vi "autonSample.vi"(0 "Auton Array":dbl[][](array[numeric]), 5 "MeasuredHeading":dbl, 9 "EncoderDistance":dbl) -> (4 "Left Drive":dbl(knob) scale=-1.0..1.0, 6 "Right Drive":dbl(knob) scale=-1.0..1.0, 10 "Turret Rotation":dbl, 14 "Feeder motor":dbl, 15 "Shooter motor output":dbl)   [LabVIEW 2011]
uses:
  Robot Global Data.vi
panel:
  in  "ShooterDesRate 2":dbl
  in  "ShooterEncRate 2":dbl
  in  "ShooterDesRate":dbl
  in  "ShooterEncRate":dbl
  in  "Balls Fired 2":i32
  in  "Balls Fired":i32
  out "Tzero":i64
  out "AccumDist":dbl
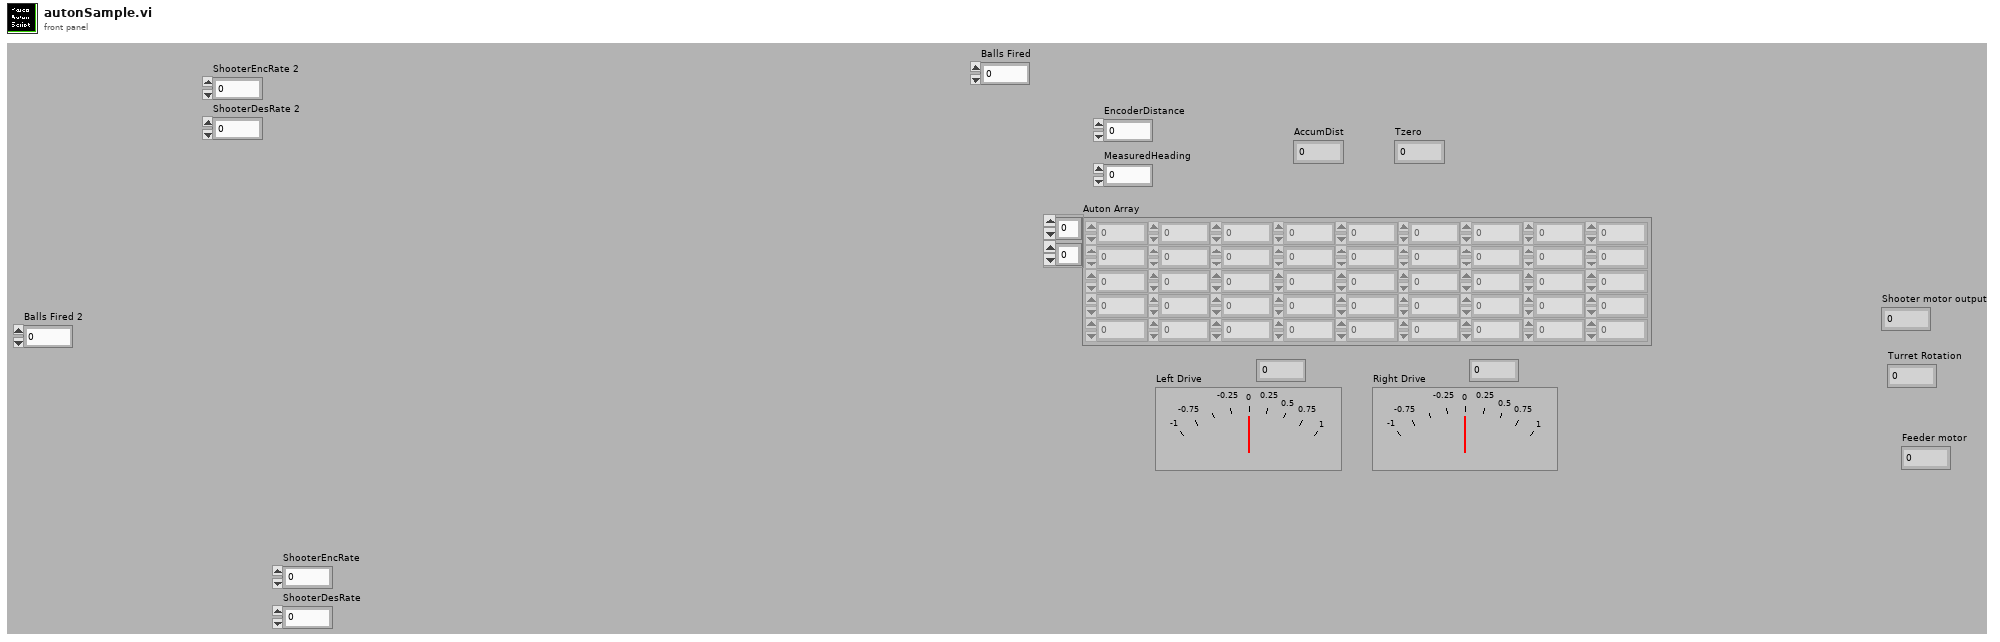
[diagram p1: front panel]
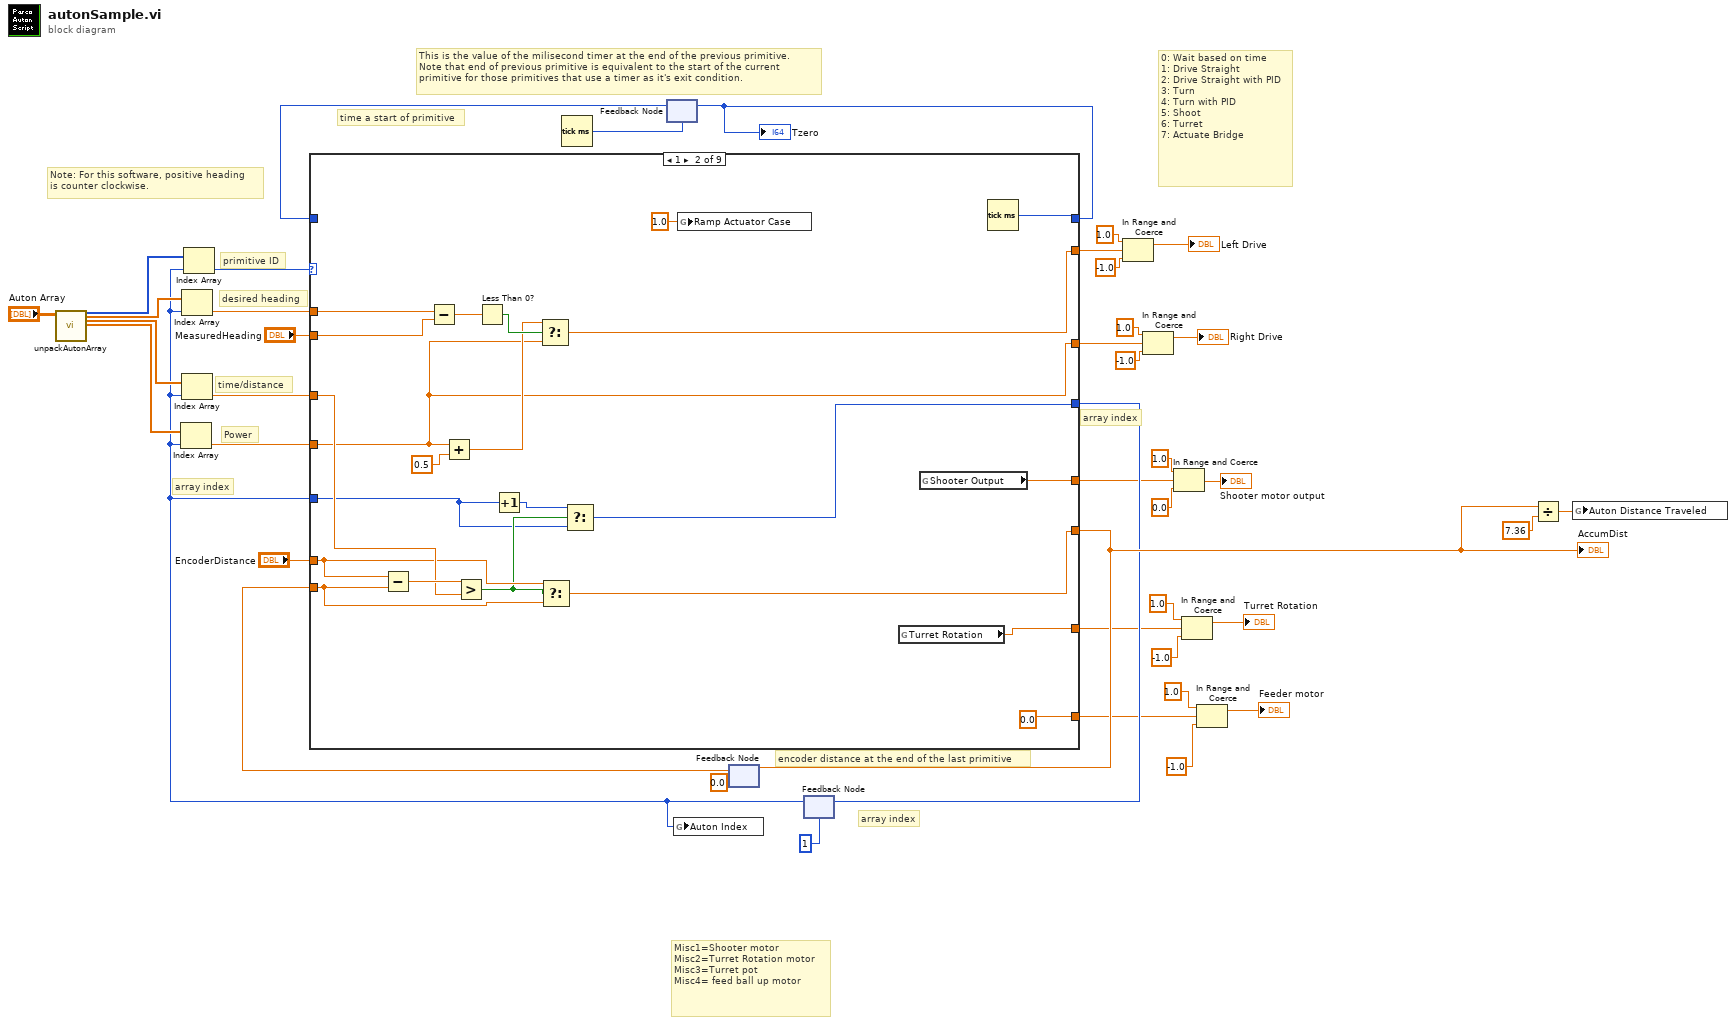
[diagram p0: block diagram]
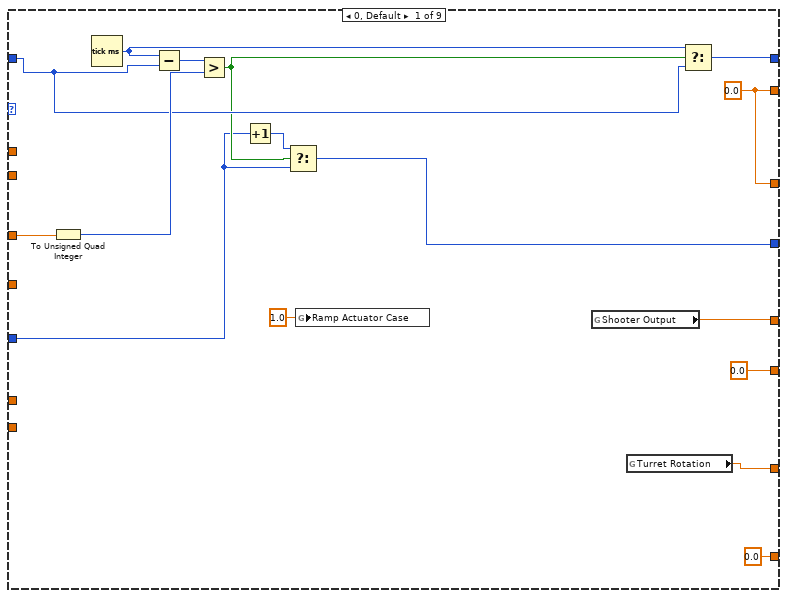
[diagram p2: hidden frame]
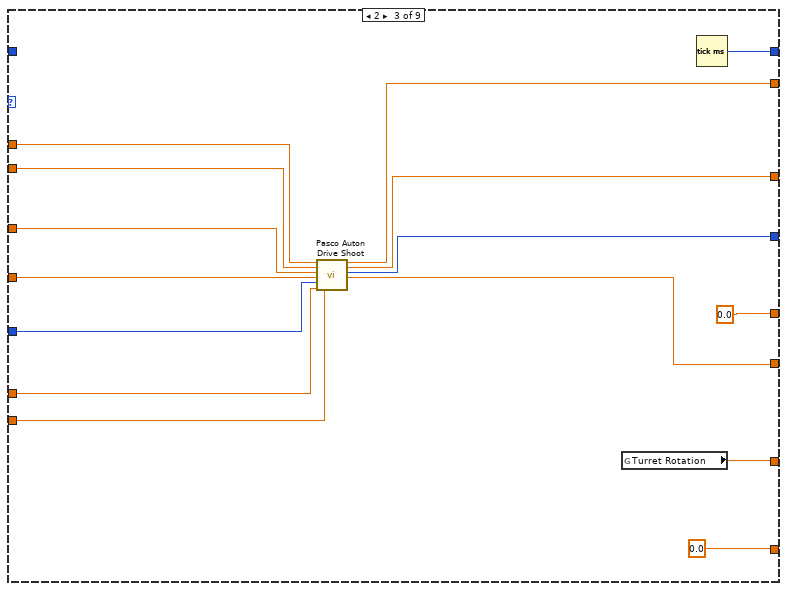
[diagram p3: hidden frame]
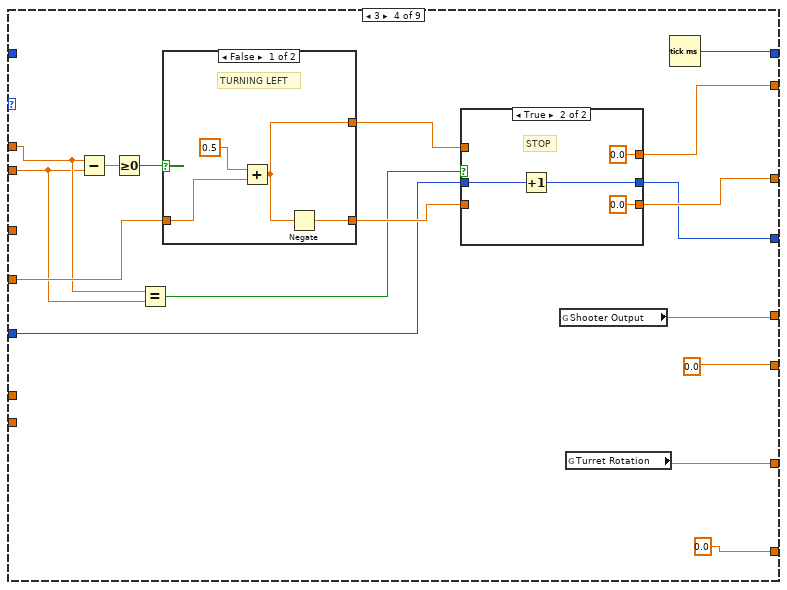
[diagram p4: hidden frame]
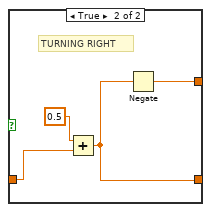
[diagram p6: hidden frame]
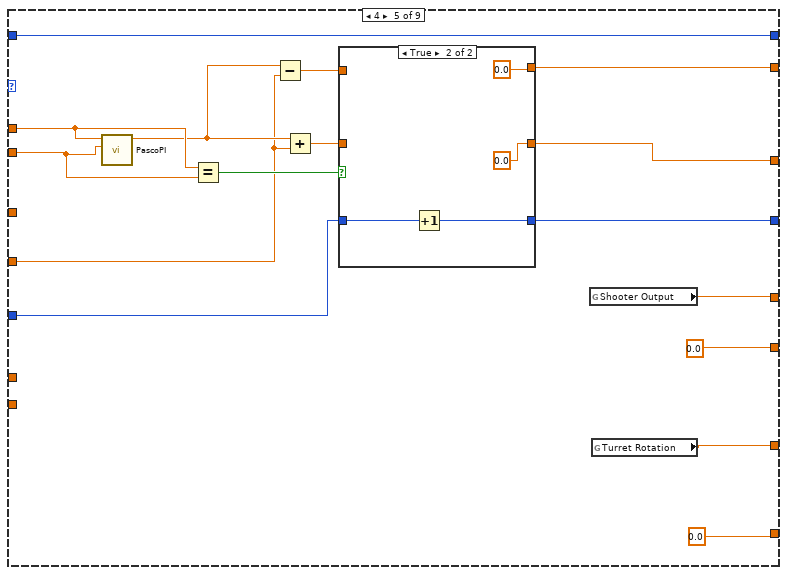
[diagram p7: hidden frame]
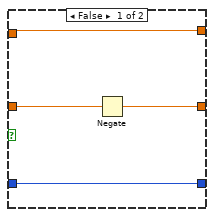
[diagram p8: hidden frame]
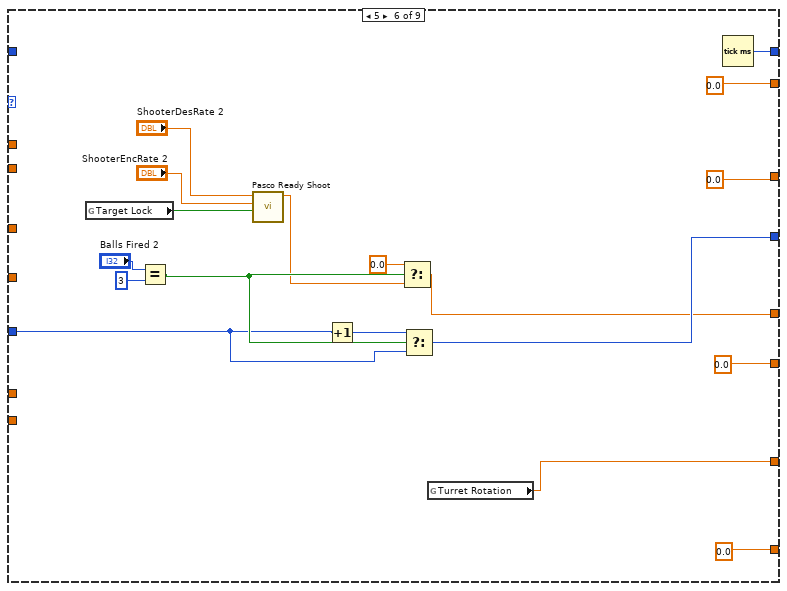
[diagram p9: hidden frame]
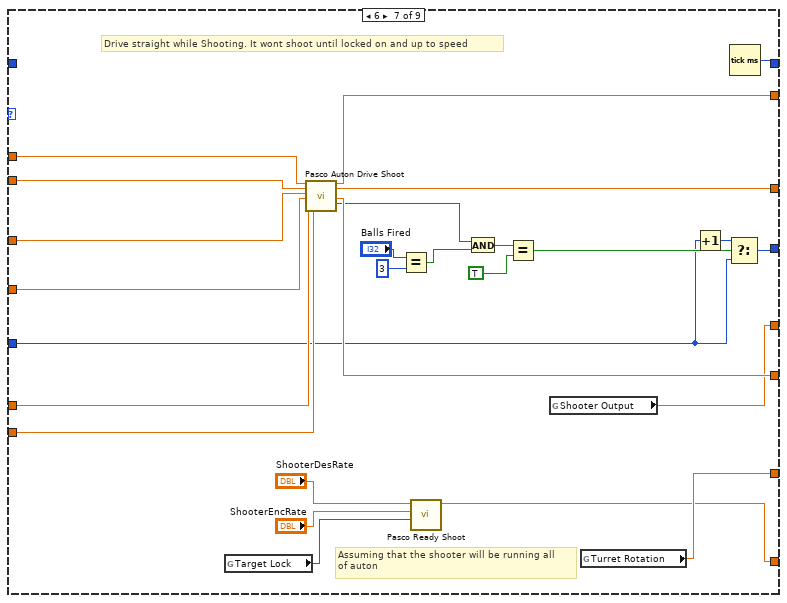
[diagram p10: hidden frame]
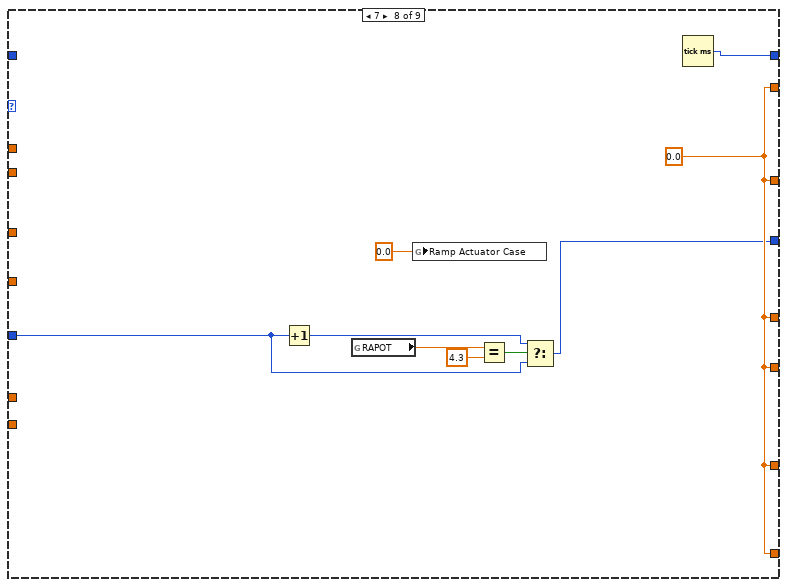
[diagram p11: hidden frame]
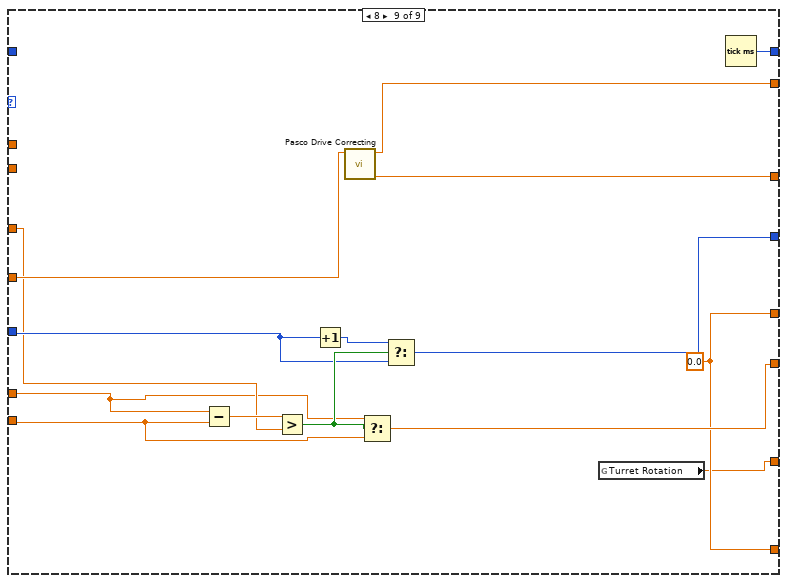
[diagram p12: hidden frame]
diagram:
  # "Misc1=Shooter motor\nMisc2=Turret Rotation motor\nMisc3=Turret pot\nMisc4= feed ball up motor"
  # "0: Wait based on time\n1: Drive Straight\n2: Drive Straight with PID\n3: Turn\n4: Turn with PID\n5: Shoot\n6: Turret\n7: Actuate Bridge"
  # "encoder distance at the end of the last primitive"
  # "Note: For this software, positive heading\nis counter clockwise."
  # "time a start of primitive"
  # "array index"
  # "array index"
  # "This is the value of the milisecond timer at the end of the previous primitive.\nNote that end of previous primitive is equivalent to the start of the current\nprimitive for those primitives that use a timer as it's exit condition."
  # "Power"
  # "array index"
  # "desired heading"
  # "primitive ID"
  # "time/distance"
  n1 = call "unpackAutonArray.vi"("all rows"="Auton Array") -> ("Primitive"=w41:i16[], "Heading"=w23:dbl[], "Distance/Time"=w24:dbl[], "Power"=w21:dbl[])  [unwired: 1 in, 22 out]
  n2 = Tick Count (ms)() -> (millisecond timer value=w35:u32)
  n3 = feedback #1(w35) -> (w39:u32)
  n4 = feedback #2(0.0 ("EncoderDistance")) -> (w20:dbl)
  n5 = feedback #3(1) -> (w2:i32)
  n6 = Index Array(array=w21, index=w2) -> (element=w37:dbl)
  n7 = Index Array(array=w23, index=w2) -> (element=w22:dbl)
  n8 = Index Array(array=w24, index=w2) -> (element=w38:dbl)
  n9 = Index Array(array=w41, index=w2) -> (element=w40:i16)
  n10 = case shown="1" w40 {
    tunnel: [w47 w65 w83 w101 w139 w163 w180 w196 w207] -> w15
    tunnel: w2 -> [w48 w66 w88 w100 w138 w156 w176 w197 w212]
    tunnel: [w58 w64 w94 w107 w143 w164 w174 w204 w216] -> w25
    tunnel: w39 -> [w54 _ _ _ w143 _ _ _ _]
    tunnel: w38 -> [w56 w73 w90 _ _ _ w193 _ w211]
    tunnel: w22 -> [_ w79 w92 w109 w133 _ w195 _ _]
    tunnel: [w46 w75 w85 w103 w140 0.0 w189 w203 w218] -> w33
    tunnel: [w46 w61 w84 w106 w141 0.0 w188 w203 w217] -> w26
    tunnel: w37 -> [_ w61 w89 w111 w130 _ w192 _ w219]
    tunnel: "EncoderDistance" -> [_ w72 w87 _ _ _ w191 _ w209]
    tunnel: "MeasuredHeading" -> [_ w78 w91 w108 w134 _ w194 _ _]
    tunnel: [0.0 ("Encoder total") w69 w82 0.0 0.0 0.0 w187 w203 w208] -> w17
    tunnel: w20 -> [_ w71 w86 _ _ _ w190 _ w210]
    tunnel: [w44 w60 0.0 ("Misc1  OUT") w96 w128 w162 w175 w203 w206] -> w11
    tunnel: [w45 w70 w81 w97 w129 w165 w178 w203 w205] -> w7
    tunnel: [0.0 ("Misc4 OUT") 0.0 0.0 0.0 0.0 0.0 w173 w203 w206] -> w3
    frame 0, Default {
      w46 = 0.0 ("Numeric")
      n11 = To Unsigned Quad Integer(1:w56) -> (0:w55:u64)
      n12 = Tick Count (ms)() -> (millisecond timer value=w53:u32)
      n13 = Subtract(x=w53, y=w54) -> (x-y=w57:u32)
      n14 = Greater?(x=w57, y=w55) -> (0:w50:bool)
      n15 = Increment(x=w48) -> (x+1=w49:i32)
      n16 = Select(t=w49, s=w50, f=w48) -> (s? t:f=w47:i32)
      n17 = global write "Robot Global Data.vi" "Ramp Actuator Case"(1.0 ("Ramp Actuator Case")) -> ()
      n18 = global read "Robot Global Data.vi" "Shooter Output"() -> (w44:dbl)
      n19 = global read "Robot Global Data.vi" "Turret Rotation"() -> (w45:dbl)
      n20 = Select(t=w53, s=w50, f=w54) -> (s? t:f=w58:u32)
    }
    frame 1 {
      n21 = Subtract(x=w72, y=w71) -> (x-y=w74:dbl)
      n22 = Subtract(x=w79, y=w78) -> (x-y=w63:dbl)
      n23 = Add(x=w61, y=0.5) -> (x+y=w62:dbl)
      n24 = Greater?(x=w74, y=w73) -> (0:w68:bool)
      n25 = Less Than 0?(x=w63) -> (x < 0?=w77:bool)
      n26 = Increment(x=w66) -> (x+1=w67:i32)
      n27 = Select(t=w62, s=w77, f=w61) -> (s? t:f=w75:dbl)
      n28 = Select(t=w72, s=w68, f=w71) -> (s? t:f=w69:dbl)
      n29 = Select(t=w67, s=w68, f=w66) -> (s? t:f=w65:i32)
      n30 = global write "Robot Global Data.vi" "Ramp Actuator Case"(1.0 ("Ramp Actuator Case")) -> ()
      n31 = global read "Robot Global Data.vi" "Turret Rotation"() -> (w70:dbl)
      n32 = global read "Robot Global Data.vi" "Shooter Output"() -> (w60:dbl)
      n33 = Tick Count (ms)() -> (millisecond timer value=w64:u32)
    }
    frame 2 {
      n34 = call "Pasco Auton Drive Shoot.vi"("Desired Heading"=w92, "Actual Heading"=w91, "time/distance"=w90, "Power"=w89, "Array"=w88, "Encoder total"=w87, "Encoder Return"=w86) -> ("Left Drive"=w85:dbl, "Right Drive"=w84:dbl, "Array Out"=w83:i32, "Encoder total"=w82:dbl)  [unwired: 8 in, 1 out]
      n35 = global read "Robot Global Data.vi" "Turret Rotation"() -> (w81:dbl)
      n36 = Tick Count (ms)() -> (millisecond timer value=w94:u32)
    }
    frame 3 {
      n37 = Subtract(x=w109, y=w108) -> (x-y=w112:dbl)
      n38 = Greater Or Equal To 0?(x=w112) -> (x >= 0?=w110:bool)
      n39 = Equal?(x=w109, y=w108) -> (x = y?=w102:bool)
      n40 = case shown="False" w110 {
        tunnel: w111 -> [w122 w124]
        tunnel: [w120 w126] -> w104
        tunnel: [w121 w125] -> w105
        frame False {
          # "TURNING LEFT"
          n41 = Add(x=0.5, y=w122) -> (x+y=w120:dbl)
          n42 = Negate(x=w120) -> (-x=w121:dbl)
        }
        frame True {
          # "TURNING RIGHT"
          n43 = Add(x=0.5, y=w124) -> (x+y=w125:dbl)
          n44 = Negate(x=w125) -> (-x=w126:dbl)
        }
      }
      n45 = case shown="True" w102 {
        tunnel: w100 -> [w115 w119]
        tunnel: [w115 w118] -> w101
        tunnel: [w114 0.0] -> w106
        tunnel: w105 -> [w114 _]
        tunnel: [w113 0.0] -> w103
        tunnel: w104 -> [w113 _]
        frame False {
          # "DRIVE"
        }
        frame True {
          # "STOP"
          n46 = Increment(x=w119) -> (x+1=w118:i32)
        }
      }
      n47 = global read "Robot Global Data.vi" "Shooter Output"() -> (w96:dbl)
      n48 = global read "Robot Global Data.vi" "Turret Rotation"() -> (w97:dbl)
      n49 = Tick Count (ms)() -> (millisecond timer value=w107:u32)
    }
    frame 4 {
      n50 = call "PascoPI.vi"("Feedback"=w134, "Setpoint"=w133) -> ("Motor Output"=w132:dbl)  [unwired: 9 in]
      n51 = Equal?(x=w133, y=w134) -> (x = y?=w136:bool)
      n52 = Subtract(x=w132, y=w130) -> (x-y=w135:dbl)
      n53 = Add(x=w132, y=w130) -> (x+y=w131:dbl)
      n54 = case shown="True" w136 {
        tunnel: w135 -> [w145 _]
        tunnel: [w147 0.0] -> w141
        tunnel: [w145 0.0] -> w140
        tunnel: [w146 w150] -> w139
        tunnel: w138 -> [w146 w151]
        tunnel: w131 -> [w144 _]
        frame False {
          n55 = Negate(x=w144) -> (-x=w147:dbl)
        }
        frame True {
          n56 = Increment(x=w151) -> (x+1=w150:i32)
        }
      }
      n57 = global read "Robot Global Data.vi" "Shooter Output"() -> (w128:dbl)
      n58 = global read "Robot Global Data.vi" "Turret Rotation"() -> (w129:dbl)
    }
    frame 5 {
      n59 = global read "Robot Global Data.vi" "Target Lock"() -> (w155:bool)
      n60 = Equal?(x="Balls Fired 2", y=3) -> (x = y?=w159:bool)
      n61 = call "Pasco Ready Shoot.vi"("Light On/Locked On"=w155, "ShooterEncRate"="ShooterEncRate 2", "ShooterDesRate"="ShooterDesRate 2") -> ("Feeder Output"=w152:dbl)  [unwired: 8 in]
      n62 = Increment(x=w156) -> (x+1=w157:i32)
      n63 = Select(t=0.0, s=w159, f=w152) -> (s? t:f=w162:dbl)
      n64 = Select(t=w157, s=w159, f=w156) -> (s? t:f=w163:i32)
      n65 = global read "Robot Global Data.vi" "Turret Rotation"() -> (w165:dbl)
      n66 = Tick Count (ms)() -> (millisecond timer value=w164:u32)
    }
    frame 6 {
      # "Drive straight while Shooting. It wont shoot until locked on and up to speed"
      # "Assuming that the shooter will be running all\nof auton"
      n67 = global read "Robot Global Data.vi" "Target Lock"() -> (w170:bool)
      n68 = call "Pasco Auton Drive Shoot.vi"("Desired Heading"=w195, "Actual Heading"=w194, "time/distance"=w193, "Power"=w192, "Encoder total"=w191, "Encoder Return"=w190) -> ("Left Drive"=w189:dbl, "Right Drive"=w188:dbl, "Encoder total"=w187:dbl, "Complete?"=w186:bool)  [unwired: 9 in, 1 out]
      n69 = Equal?(x="Balls Fired", y=3) -> (x = y?=w185:bool)
      n70 = call "Pasco Ready Shoot.vi"("Light On/Locked On"=w170, "ShooterEncRate"="ShooterEncRate", "ShooterDesRate"="ShooterDesRate") -> ("Feeder Output"=w173:dbl)  [unwired: 8 in]
      n71 = And(x=w186, y=w185) -> (x .and. y?=w182:bool)
      n72 = Equal?(x=w182, y=TRUE) -> (x = y?=w177:bool)
      n73 = global read "Robot Global Data.vi" "Shooter Output"() -> (w175:dbl)
      n74 = global read "Robot Global Data.vi" "Turret Rotation"() -> (w178:dbl)
      n75 = Increment(x=w176) -> (x+1=w179:i32)
      n76 = Select(t=w179, s=w177, f=w176) -> (s? t:f=w180:i32)
      n77 = Tick Count (ms)() -> (millisecond timer value=w174:u32)
    }
    frame 7 {
      w203 = 0.0
      n78 = Increment(x=w197) -> (x+1=w198:i32)
      n79 = global read "Robot Global Data.vi" "RAPOT"() -> (w201:dbl)
      n80 = global write "Robot Global Data.vi" "Ramp Actuator Case"(0.0 ("Auton Distance Traveled")) -> ()
      n81 = Equal?(x=w201, y=4.3) -> (x = y?=w199:bool)
      n82 = Select(t=w198, s=w199, f=w197) -> (s? t:f=w196:i32)
      n83 = Tick Count (ms)() -> (millisecond timer value=w204:u32)
    }
    frame 8 {
      w206 = 0.0
      n84 = Subtract(x=w209, y=w210) -> (x-y=w213:dbl)
      n85 = Greater?(x=w213, y=w211) -> (0:w214:bool)
      n86 = Increment(x=w212) -> (x+1=w215:i32)
      n87 = call "Pasco Drive Correcting.vi"("Power"=w219) -> ("RightDriveOutput"=w217:dbl, "LeftDriveOutput"=w218:dbl)  [unwired: 9 in]
      n88 = Select(t=w209, s=w214, f=w210) -> (s? t:f=w208:dbl)
      n89 = Select(t=w215, s=w214, f=w212) -> (s? t:f=w207:i32)
      n90 = global read "Robot Global Data.vi" "Turret Rotation"() -> (w205:dbl)
      n91 = Tick Count (ms)() -> (millisecond timer value=w216:u32)
    }
  }
  "AccumDist" <- w17
  "Tzero" <- w25
  n92 = feedback-in #1(w25) -> ()
  n93 = global write "Robot Global Data.vi" "Auton Index"(w2) -> ()
  n94 = feedback-in #2(w17) -> ()
  n95 = feedback-in #3(w15) -> ()
  n96 = In Range and Coerce(upper limit=1.0, x=w33, lower limit=-1.0) -> (coerced(x)=→"Left Drive":dbl)  [unwired: 1 out]
  n97 = In Range and Coerce(upper limit=1.0, x=w26, lower limit=-1.0) -> (coerced(x)=→"Right Drive":dbl)  [unwired: 1 out]
  n98 = In Range and Coerce(upper limit=1.0, x=w11, lower limit=0.0) -> (coerced(x)=→"Shooter motor output":dbl)  [unwired: 1 out]
  n99 = In Range and Coerce(upper limit=1.0, x=w7, lower limit=-1.0) -> (coerced(x)=→"Turret Rotation":dbl)  [unwired: 1 out]
  n100 = In Range and Coerce(upper limit=1.0, x=w3, lower limit=-1.0) -> (coerced(x)=→"Feeder motor":dbl)  [unwired: 1 out]
  n101 = Divide(x=w17, y=7.36) -> (x/y=w1:dbl)
  n102 = global write "Robot Global Data.vi" "Auton Distance Traveled"(w1) -> ()
